vi "Menu.vi"() -> ()   [LabVIEW 2017]
panel:
  out "String":string
  in  "??":bool
  in  "?":bool
  in  "Highball":bool
  in  "Jack & Coke":bool
  # "Cocktails Menu"
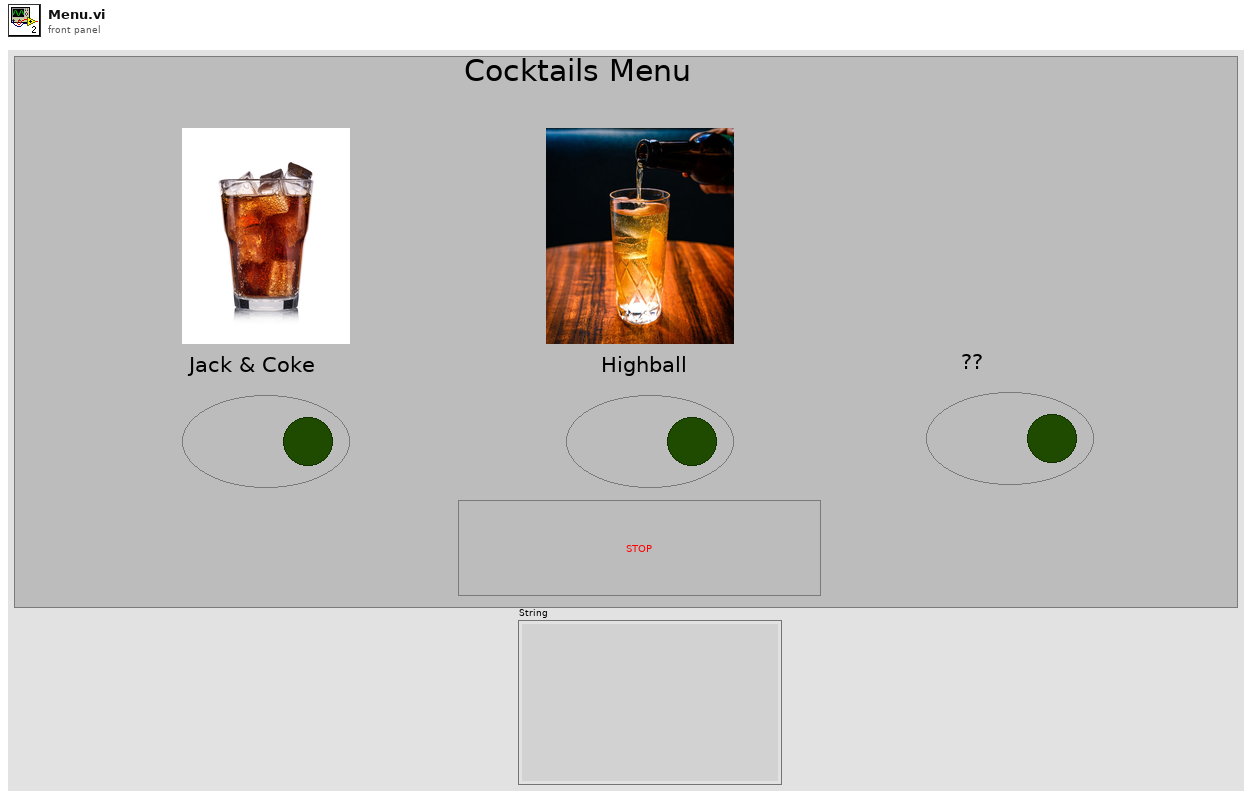
[diagram p1: front panel]
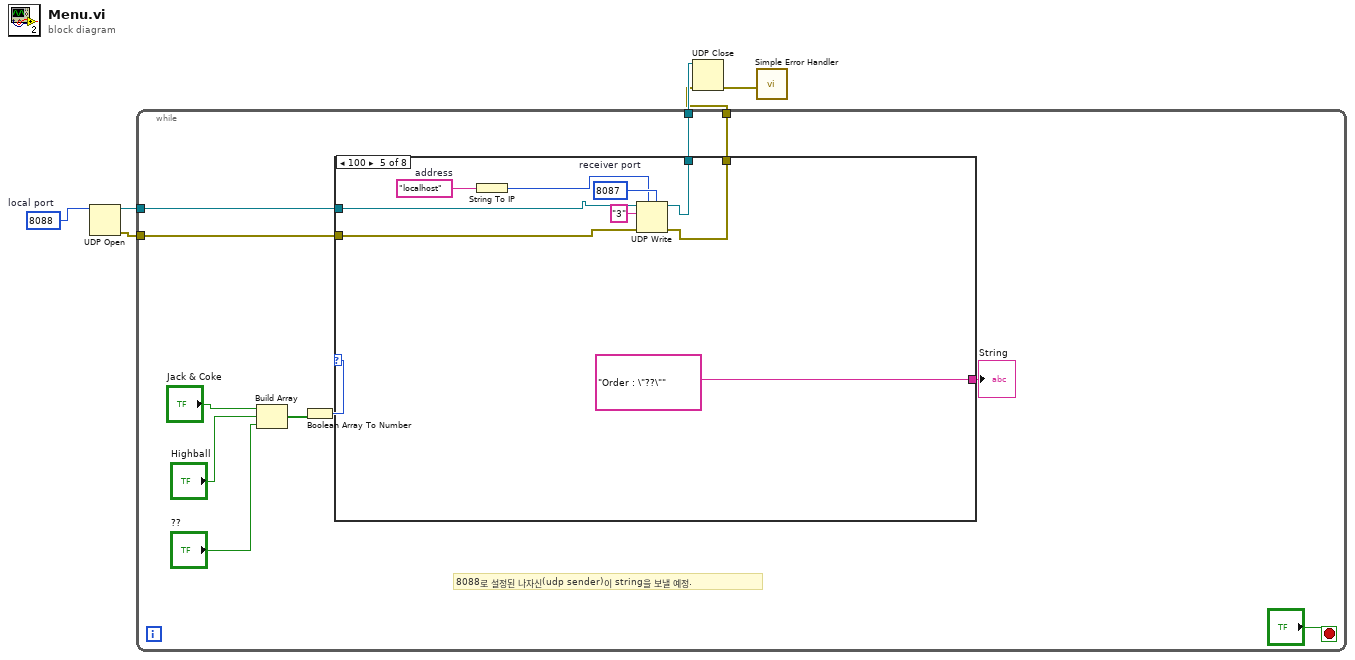
[diagram p0: block diagram]
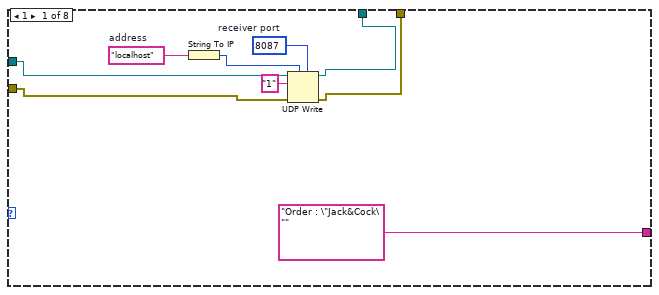
[diagram p2: hidden frame]
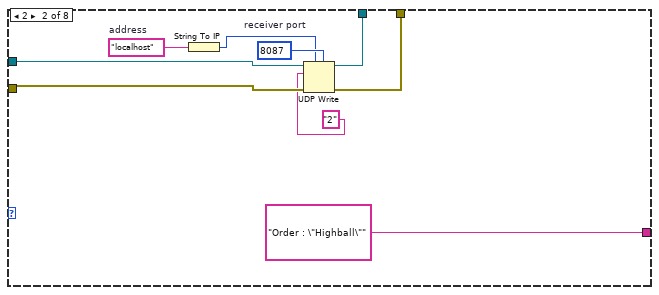
[diagram p3: hidden frame]
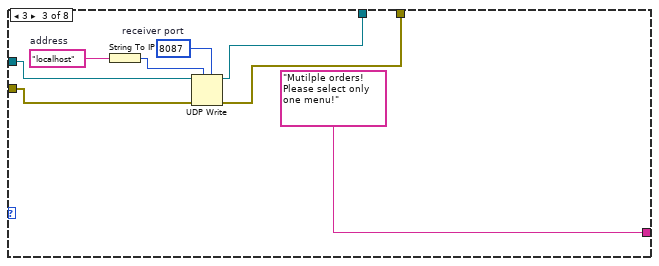
[diagram p4: hidden frame]
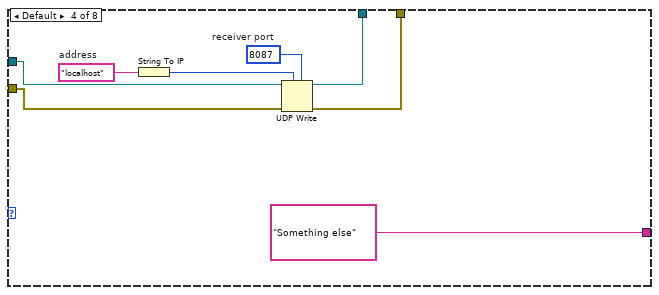
[diagram p5: hidden frame]
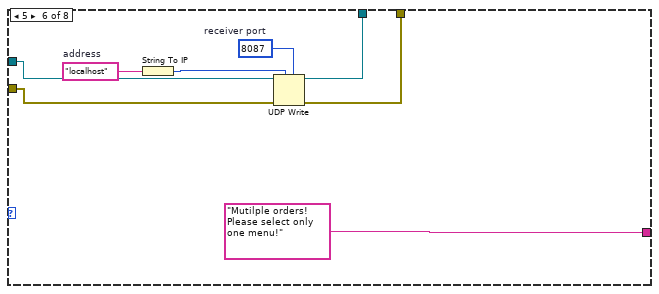
[diagram p6: hidden frame]
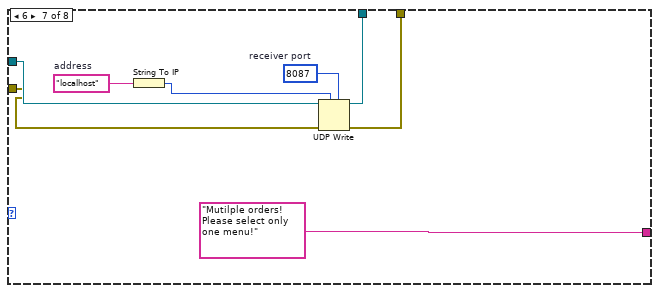
[diagram p7: hidden frame]
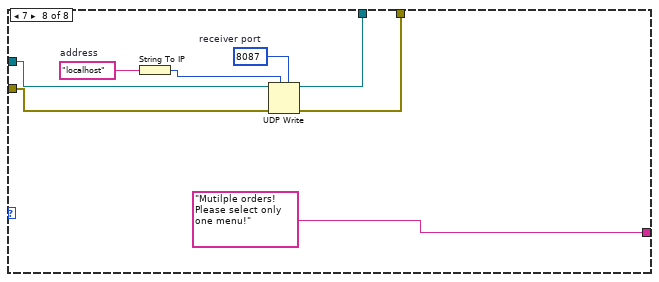
[diagram p8: hidden frame]
diagram:
  w6 = u16 8088  # local port
  n1 = UDP Open(11:w6) -> (port=w2:refnum<k16>, 0:w1:errorcluster)  [unwired: 4 in, 1 out]
  n2 = while {
    tunnel: [w10] -> w4
    tunnel: [w9] -> w3
    tunnel: w2 -> [w8]
    tunnel: w1 -> [w7]
    stop <- "?" stop-if-true
    # "8088로 설정된 나자신(udp sender)이 string을 보낼 예정."
    n3 = Build Array("Jack & Coke", "Highball", "??") -> (w15:bool[])
    n4 = Boolean Array To Number(Boolean array=w15) -> (number=w11:u32)
    n5 = case shown="100" w11 {
      tunnel: ["Order : \"Jack&Cock\"" "Order : \"Highball\"" "Mutilple orders! Please select only one menu!" "Something else" "Order : \"??\"" "Mutilple orders! Please select only one menu!" "Mutilple orders! Please select only one menu!" "Mutilple orders! Please select only one menu!"] -> w13
      tunnel: [w22 w31 w39 w47 w58 w64 w72 w80] -> w10
      tunnel: [w21 w30 w38 w46 w57 w63 w71 w79] -> w9
      tunnel: w8 -> [w24 w33 w41 w49 w56 w66 w74 w82]
      tunnel: w7 -> [w23 w32 w40 w48 w55 w65 w73 w81]
      frame 1 {
        w20 = "localhost"  # address
        w25 = u16 8087  # receiver port
        n6 = String To IP(1:w20) -> (0:w19:u32)
        n7 = UDP Write(address=w19, port or service name=w25, connection ID=w24, data in="1", 8:w23) -> (error out=w21:errorcluster, 3:w22:refnum<k16>)  [unwired: 1 in]
      }
      frame 2 {
        w29 = "localhost"  # address
        w34 = u16 8087  # receiver port
        n8 = String To IP(1:w29) -> (0:w28:u32)
        n9 = UDP Write(address=w28, port or service name=w34, connection ID=w33, data in="2", 8:w32) -> (error out=w30:errorcluster, 3:w31:refnum<k16>)  [unwired: 1 in]
      }
      frame 3 {
        w37 = "localhost"  # address
        w42 = u16 8087  # receiver port
        n10 = String To IP(1:w37) -> (0:w36:u32)
        n11 = UDP Write(address=w36, port or service name=w42, connection ID=w41, 8:w40) -> (error out=w38:errorcluster, 3:w39:refnum<k16>)  [unwired: 2 in]
      }
      frame Default {
        w45 = "localhost"  # address
        w50 = u16 8087  # receiver port
        n12 = String To IP(1:w45) -> (0:w44:u32)
        n13 = UDP Write(address=w44, port or service name=w50, connection ID=w49, 8:w48) -> (error out=w46:errorcluster, 3:w47:refnum<k16>)  [unwired: 2 in]
      }
      frame 4 {
        w54 = "localhost"  # address
        w59 = u16 8087  # receiver port
        n14 = String To IP(1:w54) -> (0:w53:u32)
        n15 = UDP Write(address=w53, port or service name=w59, connection ID=w56, data in="3", 8:w55) -> (error out=w57:errorcluster, 3:w58:refnum<k16>)  [unwired: 1 in]
      }
      frame 5 {
        w62 = "localhost"  # address
        w67 = u16 8087  # receiver port
        n16 = String To IP(1:w62) -> (0:w61:u32)
        n17 = UDP Write(address=w61, port or service name=w67, connection ID=w66, 8:w65) -> (error out=w63:errorcluster, 3:w64:refnum<k16>)  [unwired: 2 in]
      }
      frame 6 {
        w70 = "localhost"  # address
        w75 = u16 8087  # receiver port
        n18 = String To IP(1:w70) -> (0:w69:u32)
        n19 = UDP Write(address=w69, port or service name=w75, connection ID=w74, 8:w73) -> (error out=w71:errorcluster, 3:w72:refnum<k16>)  [unwired: 2 in]
      }
      frame 7 {
        w78 = "localhost"  # address
        w83 = u16 8087  # receiver port
        n20 = String To IP(1:w78) -> (0:w77:u32)
        n21 = UDP Write(address=w77, port or service name=w83, connection ID=w82, 8:w81) -> (error out=w79:errorcluster, 3:w80:refnum<k16>)  [unwired: 2 in]
      }
    }
    "String" <- w13
  }
  n22 = UDP Close(connection ID=w4, 8:w3) -> (error out=w5:errorcluster)  [unwired: 1 out]
  n23 = call <vilib>:"Simple Error Handler.vi"("error in (no error)"=w5) -> ()  [unwired: 4 in, 5 out]
